vi "ATF-Pump-DO Start.vi"(8 "error in":errorcluster, 9 "DO config":T1(array[cluster]), 11 "Refnum in":refnum<k21>) -> (0 "error out":errorcluster, 3 "Refnum out":refnum<k21>)   [LabVIEW 2022 SP3]
doc: "This VI is for start for Analog Output"
uses:
  RT Controls/ATF-Pump-FGV Read write.ctl
panel:
  out "Array":bool[](array[boolean])
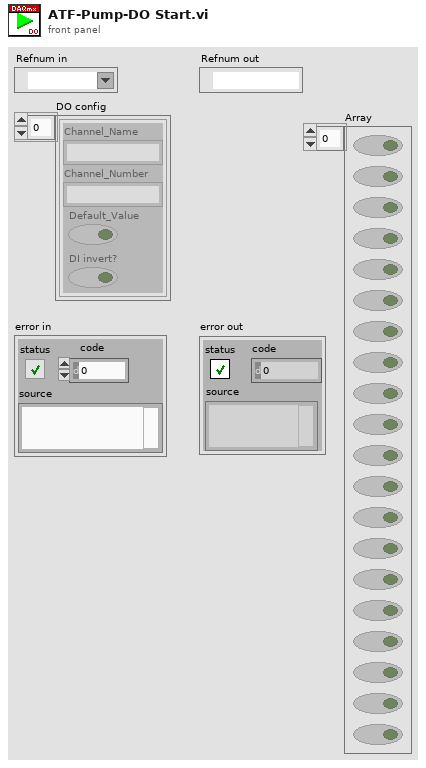
[diagram p1: front panel]
types:
  T1 = cluster{"Channel_Name":string, "Channel_Number":string, "Default_Value":bool, "DI invert?":bool}[]
  T2 = enum16{"Init", "Read", "Write 'All'", "Write 'n'", "Write Safe Value", "Write Start Time", "Overwrite Pattern", "Overwrite Pattern with Start", "Append Pattern", "Start Pattern Mode", "Abort Pattern Mode", "Read 1"}
  T3 = typedef "ATF-Pump-FGV Read write.ctl" = enum16{"Write", "Read"}
  T4 = cluster{"Samples to Read":i32, "Pattern Mode?":bool, "dt(sec)":dbl, "DO Init Time (Samples)":i32, "dt per Read/Write":dbl, "Write Pointer":i32, "Pattern Size":i32, "Loop Rate (mSec)":i32, "Buffer Size (Samples)":i32, "Sampling rate":dbl, "Max DO Delay Time (samples)":dbl, "Min DO Delay Time (samples)":dbl, "Queue Size":i32, "DO Init Sample Duration (Sec)":dbl}
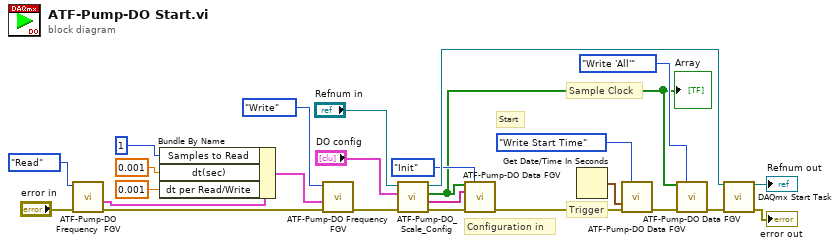
[diagram p0: block diagram]
diagram:
  # "Start"
  # "Trigger"
  # "Sample Clock"
  # "Configuration in"
  n1 = call "ATF-Pump-DO Frequency  FGV.vi"("error in"="error in", "Write/Read"=ATF-Pump-FGV_Read_write."Read") -> ("error in 2"=w8:errorcluster, "DO Set Frequency (R)"=w14:T4)  [unwired: 8 in]
  n2 = Bundle By Name(cluster=w14, "Samples to Read"=1, "dt(sec)"=0.001, "dt per Read/Write"=0.001) -> (w13:T4)
  n3 = call "ATF-Pump-DO Frequency  FGV.vi"("error in"=w8, "DO Set Frequency (W)"=w13, "Write/Read"=ATF-Pump-FGV_Read_write."Write") -> ("error in 2"=w7:errorcluster)  [unwired: 7 in, 1 out]
  n4 = call "ATF-Pump-DO_Scale_Config.vi"("error in (no error)"=w7, "DO config"="DO config", "Refnum in"="Refnum in") -> ("error out"=w6:errorcluster, "Array 2"=w20:string[], "Array"=w2:bool[], "Refnum out"=w24:refnum<k21>)  [unwired: 5 in]
  "Array" <- w2
  n5 = call "ATF-Pump-DO Data FGV.vi"("DO Values In"=w2, "Option"=T2."Init", "DO Channel Names"=w20, "error in (no error)"=w6) -> ("error out"=w17:errorcluster)  [unwired: 5 in, 6 out]
  n6 = Get Date/Time In Seconds() -> (seconds since 1Jan1904=w18:timestamp)
  n7 = call "ATF-Pump-DO Data FGV.vi"("Option"=T2."Write Start Time", "Time Stamp In"=w18, "error in (no error)"=w17) -> ("error out"=w1:errorcluster)  [unwired: 6 in, 6 out]
  n8 = call "ATF-Pump-DO Data FGV.vi"("DO Values In"=w2, "Option"=T2."Write 'All'", "error in (no error)"=w1) -> ("error out"=w4:errorcluster)  [unwired: 6 in, 6 out]
  n9 = call <vilib>:"DAQmx Start Task.vi"("task/channels in"=w24, "error in"=w4) -> ("task out"=→"Refnum out":refnum<k21>, "error out"=→"error out":errorcluster)  [unwired: 12 in]
